vi "Color Match.vi"   [LabVIEW 2019]
uses:
  Framework/Robot Global Data.vi
types:
  T1 = typedef "Color Sensor V3 DevRef.ctl" = cluster{"I2CDevRef":T2}
  T2 = typedef "WPI_I2CDevRef.ctl" = cluster{"DevStatus":errorcluster, "Device Address":u8, "Handle":i32, "I2C Bus":T3}
  T3 = typedef "i2c_bus.ctl" = enum16{"I2C On-Board", "I2C MXP", "Invalid"}
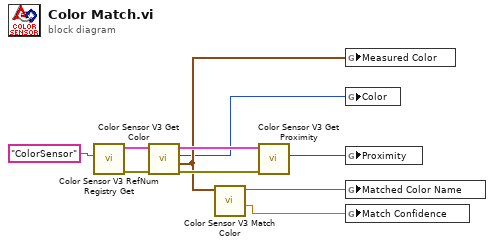
[diagram p0: block diagram]
diagram:
  n1 = call <vilib>:"Color Sensor V3 RefNum Registry Get.vi"("refnum name"="ColorSensor") -> ("error out"=w8:errorcluster, "ColorSensorDevRef"=w7:T1)  [unwired: 9 in]
  n2 = call <vilib>:"Color Sensor V3 Get Color.vi"("error in (no error)"=w8, "ColorSensorDevRef"=w7) -> ("error out"=w10:errorcluster, "Normalized Color"=w5:cluster{"R":dbl, "G":dbl, "B":dbl}, "Color"=w4:u32, "ColorSensorDevRef out"=w9:T1)  [unwired: 6 in]
  n3 = call <vilib>:"Color Sensor V3 Match Color.vi"("Measured Color"=w5) -> ("Confidence"=w1:dbl, "Matched Color Name"=w2:string)  [unwired: 8 in, 1 out]
  n4 = call <vilib>:"Color Sensor V3 Get Proximity.vi"("error in (no error)"=w10, "ColorSensorDevRef"=w9) -> ("Proximity"=w3:u16)  [unwired: 7 in, 2 out]
  n5 = global write "Robot Global Data.vi" "Measured Color"(w5) -> ()
  n6 = global write "Robot Global Data.vi" "Color"(w4) -> ()
  n7 = global write "Robot Global Data.vi" "Proximity"(w3) -> ()
  n8 = global write "Robot Global Data.vi" "Matched Color Name"(w2) -> ()
  n9 = global write "Robot Global Data.vi" "Match Confidence"(w1) -> ()
